vi "MainInterface.vi"() -> ()   [LabVIEW 2014]
uses:
  State.ctl
  <vilib>/DAQmx/create/channels.llb/DAQmx Create Channel (AO-Voltage-Basic).vi
  <vilib>/DAQmx/configure/timing.llb/DAQmx Timing (Sample Clock).vi
  <vilib>/DAQmx/write.llb/DAQmx Write (Analog 1D DBL 1Chan NSamp).vi
panel:
  out "Simulation":dbl[](graph)
  in  "Timer":cluster{"Repeat?":bool, "Timer":u32} {"Timer" min=1 max=5 step=1 format="%d s"}
  in  "Signal Spec":T1={"Duration"=1, "Intensity"=100, "Rate"=10} {"Rate" min=1 max=1000 step=1 format="%d Hz"; "Intensity" max=3000 step=1 format="%d mV"; "Duration" min=1 max=100 step=1 format="%d ms"}
  in  "Output?":bool
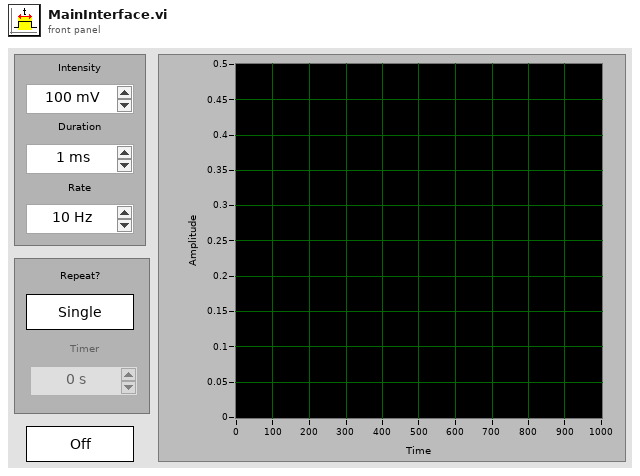
[diagram p1: front panel]
types:
  T1 = cluster{"Duration":u16, "Intensity":u16, "Rate":u16}
  T2 = typedef "State.ctl" = enum16{"Initialize", "PreRun", "Running", "Stopping", "DeInit"}
  T3 = enum8{"Enabled", "Disabled", "Disabled and Grayed Out"}
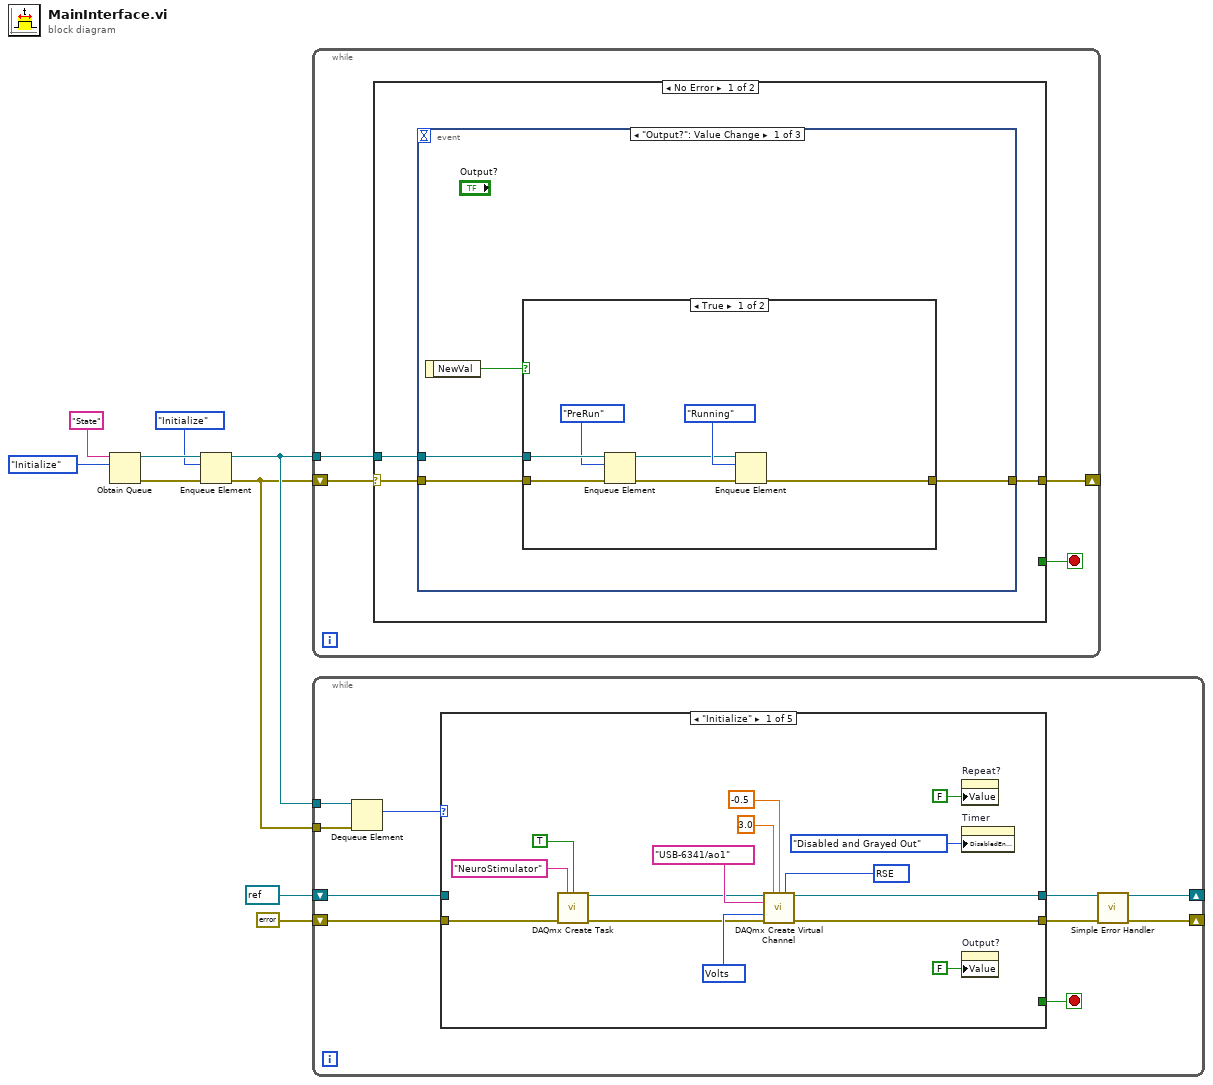
[diagram p0: block diagram]
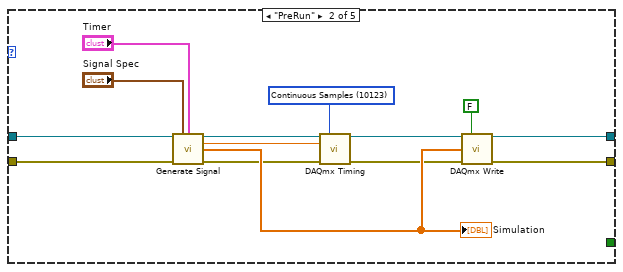
[diagram p2: hidden frame]
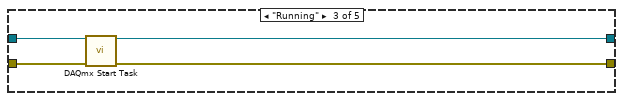
[diagram p3: hidden frame]
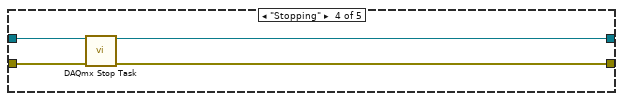
[diagram p4: hidden frame]
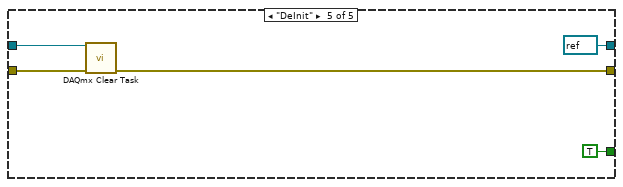
[diagram p5: hidden frame]
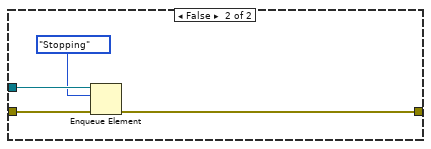
[diagram p6: hidden frame]
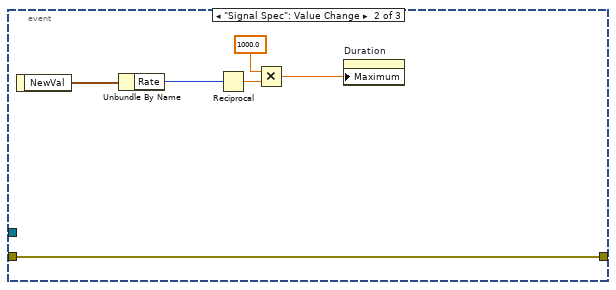
[diagram p7: hidden frame]
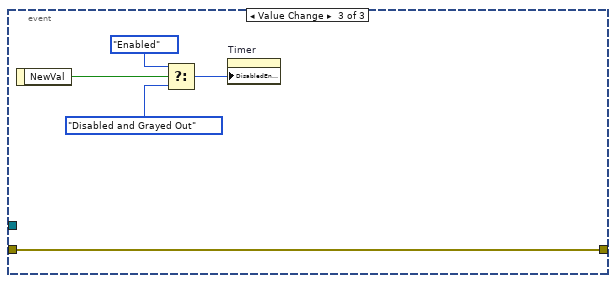
[diagram p8: hidden frame]
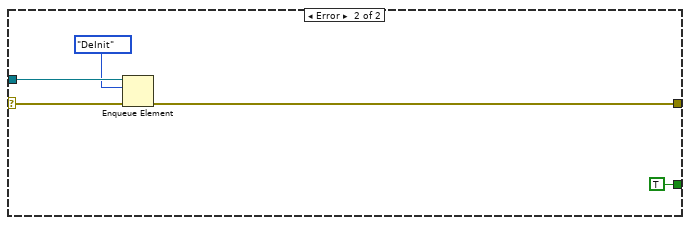
[diagram p9: hidden frame]
diagram:
  n1 = Obtain Queue(name (unnamed)="State", element data type=State."Initialize") -> (queue out=w7:refnum<queue>, error out=w3:errorcluster)  [unwired: 3 in, 1 out]
  n2 = Enqueue Element(queue=w7, element=State."Initialize", error in (no error)=w3) -> (queue out=w4:refnum<queue>, error out=w2:errorcluster)  [unwired: 1 in, 1 out]
  n3 = while {
    tunnel: w4 -> [w13]
    shift-right: [w12] -> _
    shift-left: w2 -> [w11]
    stop <- w10 stop-if-true
    n4 = case shown="No Error" w11 {
      selector: w11 -> [w14 w47]
      tunnel: w13 -> [w16 w46]
      tunnel: [w15 w44] -> w12
      tunnel: [_ TRUE] -> w10
      frame No Error {
        n5 = event shown="[0] \"Output?\": Value Change" {
          selector: _ -> [_ _ _]
          dyn-events: _ -> [_ _ _]
          timeout: _ -> [_ _ _]
          tunnel: w16 -> [w20 _ _]
          tunnel: w14 -> [w19 w34 w38]
          tunnel: [w17 w34 w38] -> w15
          event "Output?": Value Change {
            n6 = event-data() -> ("NewVal"=w18:bool)  [unwired: 1 in]
            n7 = case shown="True" w18 {
              tunnel: w20 -> [w27 w31]
              tunnel: w19 -> [w26 w30]
              tunnel: [w21 w28] -> w17
              frame True {
                n8 = Enqueue Element(queue=w27, element=State."PreRun", error in (no error)=w26) -> (queue out=w23:refnum<queue>, error out=w22:errorcluster)  [unwired: 1 in, 1 out]
                n9 = Enqueue Element(queue=w23, element=State."Running", error in (no error)=w22) -> (error out=w21:errorcluster)  [unwired: 1 in, 2 out]
              }
              frame False {
                n10 = Enqueue Element(queue=w31, element=State."Stopping", error in (no error)=w30) -> (error out=w28:errorcluster)  [unwired: 1 in, 2 out]
              }
            }
          }
          event "Signal Spec": Value Change {
            n11 = event-data() -> ("NewVal"=w37:T1)  [unwired: 1 in]
            n12 = Unbundle By Name(w37) -> ("Rate"=w36:u16)
            n13 = Reciprocal(x=w36) -> (1/x=w35:dbl)
            n14 = Multiply(x=1000.0, y=w35) -> (x*y=w33:dbl)
            n15 = property on="Duration" class="DigNum (strict)"("Maximum"=w33) -> ()  [unwired: 2 in, 2 out]
          }
          event "Timer.Repeat?": Value Change {
            n16 = event-data() -> ("NewVal"=w42:bool)  [unwired: 1 in]
            n17 = Select(t=T3."Enabled" ("Disabled"), s=w42, f=T3."Disabled and Grayed Out" ("Disabled")) -> (s? t:f=w39:T3)
            n18 = property on="Timer" class="DigNum (strict)"("DisabledEnum"=w39) -> ()  [unwired: 2 in, 2 out]
          }
        }
      }
      frame Error {
        n19 = Enqueue Element(queue=w46, element=State."DeInit", error in (no error)=w47) -> (error out=w44:errorcluster)  [unwired: 1 in, 2 out]
      }
    }
  }
  n20 = while {
    tunnel: w4 -> [w56]
    tunnel: w2 -> [w55]
    shift-right: [w52] -> _
    shift-left: refnum<k21> refnum ("task in") -> [w53]
    shift-right: [w48] -> _
    shift-left: errorcluster {"status"=FALSE, "code"=0, "source"=""} ("error out") -> [w50]
    stop <- w49 stop-if-true
    n21 = Dequeue Element(queue=w56, error in (no error)=w55) -> (element=w54:T2)  [unwired: 1 in, 3 out]
    n22 = case shown="\"Initialize\"" w54 {
      tunnel: w53 -> [_ w73 w88 w92 w97]
      tunnel: [w60 w83 w87 w90 refnum<k21> refnum ("task out")] -> w52
      tunnel: [w61 w84 w86 w91 w96] -> w51
      tunnel: w50 -> [w71 w74 w89 w93 w98]
      tunnel: [_ _ _ _ TRUE] -> w49
      frame "Initialize" {
        w57 = 10083 items=["Default"=-1, "RSE"=10083, "Differential"=10106, "Pseudodifferential"=12529] ("output terminal configuration")
        w64 = 10348 items=["Volts"=10348, "From Custom Scale"=10065] ("units")
        n23 = call <vilib>:"DAQmx Create Task.vi"("new task name"="NeuroStimulator", "auto cleanup"=TRUE, "error in"=w71) -> ("task out"=w62:refnum<k21>, "error out"=w63:errorcluster)  [unwired: 11 in]
        n24 = call-poly <vilib>:"DAQmx Create Virtual Channel.vi"("task in"=w62, "maximum value"=3.0, "minimum value"=-0.5, "output terminal configuration"=w57, "physical channels"=tag "USB-6341/ao1", "units"=w64, "error in"=w63) -> ("task out"=w60:refnum<k21>, "error out"=w61:errorcluster)  [unwired: 7 in]
        n25 = property on="Repeat?" class="Bool (strict)"("Value"=FALSE) -> ()  [unwired: 2 in, 2 out]
        n26 = property on="Timer" class="DigNum (strict)"("DisabledEnum"=T3."Disabled and Grayed Out" ("Disabled")) -> ()  [unwired: 2 in, 2 out]
        n27 = property on="Output?" class="Bool (strict)"("Value"=FALSE ("Output?")) -> ()  [unwired: 2 in, 2 out]
      }
      frame "PreRun" {
        w85 = 10123 items=["Finite Samples"=10178, "Continuous Samples"=10123, "Hardware Timed Single Point"=12522] ("sample mode")
        n28 = call "Generate Signal.vi"("task in"=w73, "Signal Spec"="Signal Spec", "Timer"="Timer", "error in (no error)"=w74) -> ("task out"=w79:refnum<k21>, "Scan Rate (Hz)"=w77:dbl, "Data"=w76:dbl[], "error out"=w75:errorcluster)  [unwired: 8 in]
        "Simulation" <- w76
        n29 = call-poly <vilib>:"DAQmx Timing.vi"("task/channels in"=w79, "sample mode"=w85, "rate"=w77, "error in"=w75) -> ("task out"=w78:refnum<k21>, "error out"=w72:errorcluster)  [unwired: 10 in]
        n30 = call-poly <vilib>:"DAQmx Write.vi"("task/channels in"=w78, "auto start"=FALSE, "data"=w76, "error in"=w72) -> ("task out"=w83:refnum<k21>, "error out"=w84:errorcluster)  [unwired: 9 in, 1 out]
      }
      frame "Running" {
        n31 = call <vilib>:"DAQmx Start Task.vi"("task/channels in"=w88, "error in"=w89) -> ("task out"=w87:refnum<k21>, "error out"=w86:errorcluster)  [unwired: 12 in]
      }
      frame "Stopping" {
        n32 = call <vilib>:"DAQmx Stop Task.vi"("task/channels in"=w92, "error in"=w93) -> ("task out"=w90:refnum<k21>, "error out"=w91:errorcluster)  [unwired: 12 in]
      }
      frame "DeInit" {
        n33 = call <vilib>:"DAQmx Clear Task.vi"("task in"=w97, "error in"=w98) -> ("error out"=w96:errorcluster)  [unwired: 13 in]
      }
    }
    n34 = call <vilib>:"Simple Error Handler.vi"("error in (no error)"=w51) -> ("error out"=w48:errorcluster)  [unwired: 4 in, 4 out]
  }
